vi "send Command Response.vi"(8 "error in (no error)":errorcluster, 11 "REx Command - Root in":refnum<class "REx Command - Root.lvclass">) -> (0 "error out":errorcluster, 3 "REx Command - Root out":refnum<class "REx Command - Root.lvclass">)   [LabVIEW 2012, in "REx.lvlib" / "REx Command - Root.lvclass"]
uses:
  REx Command - Root.lvclass
  REx Command - Root.lvclass/REx Command - Root.ctl
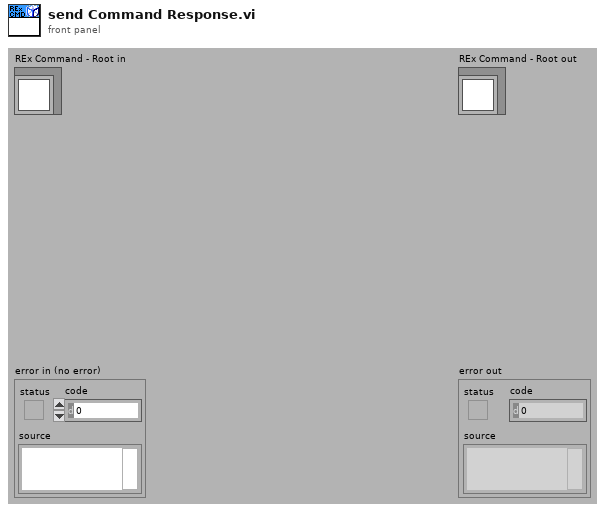
[diagram p1: front panel]
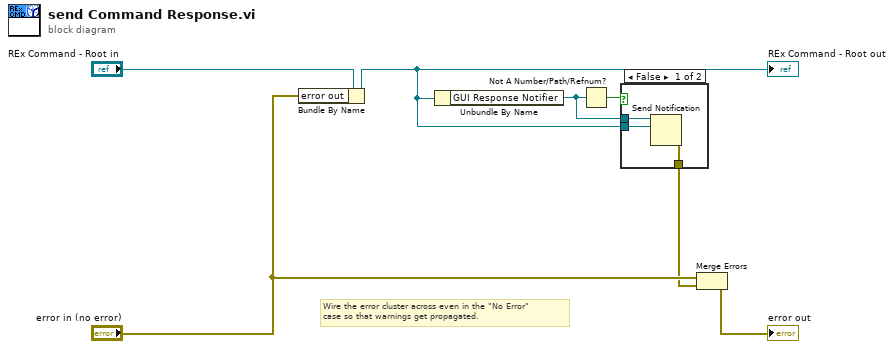
[diagram p0: block diagram]
diagram:
  # "Wire the error cluster across even in the \"No Error\"\ncase so that warnings get propagated."
  n1 = Bundle By Name(cluster="REx Command - Root in", "error out"="error in (no error)") -> (w5:refnum<class "REx Command - Root.lvclass">)
  "REx Command - Root out" <- w5
  n2 = Unbundle By Name(w5) -> ("GUI Response Notifier"=w3:refnum<notifier>)
  n3 = Not A Number/Path/Refnum?(number/path/refnum=w3) -> (NaN/Path/Refnum?=w4:bool)
  n4 = case shown="False" w4 {
    tunnel: w5 -> [w10 _]
    tunnel: w3 -> [w9 _]
    tunnel: [w8 _] -> w2
    frame False {
      n5 = Send Notification(notification=w10, notifier=w9) -> (error out=w8:errorcluster)  [unwired: 1 in, 1 out]
    }
    frame True {
    }
  }
  n6 = Merge Errors("error in (no error)", w2) -> (→"error out":errorcluster)
